vi "trio_start_home.vi"(8 "error in":errorcluster, 11 "reference in":refnum<k7>) -> (0 "Error out":errorcluster, 3 "reference out":refnum<k7>)   [LabVIEW 2024]
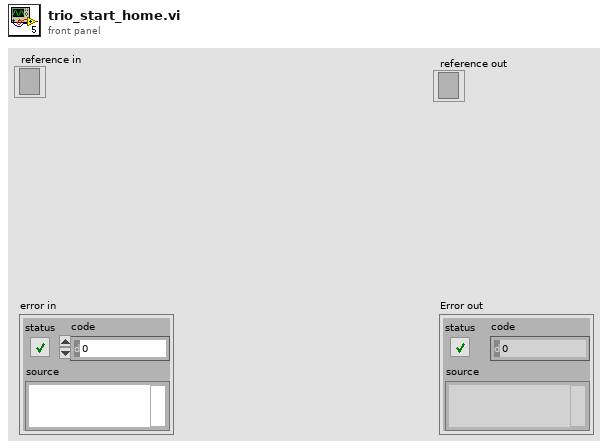
[diagram p1: front panel]
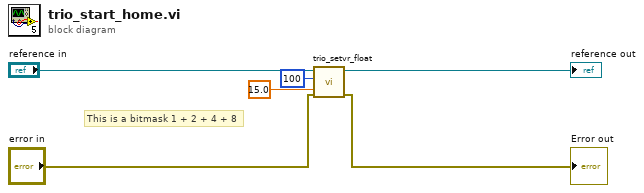
[diagram p0: block diagram]
diagram:
  # "This is a bitmask 1 + 2 + 4 + 8"
  n1 = call "trio_setvr_float.vi"("error in (no error)"="error in", "Value"=15.0, "Vr #"=i16 100, "reference in"="reference in") -> ("error out"=→"Error out":errorcluster, "reference out"=→"reference out":refnum<k7>)  [unwired: 5 in, 1 out]
